vi "cRIO_4DoF_Admittance_controller_v3.vi"(0 "F":dbl[](array[numeric]), 1 "v_2 in":dbl[](array[numeric]), 2 "c":dbl[][](array[numeric])=[[1.0, 0.0, 0.0, 0.0], [0.0, 1.0, 0.0, 0.0], [0.0, 0.0, 1.0, 0.0], [0.0, 0.0, 0.0, 0.001]], 3 "m":dbl[][](array[numeric])=[[0.4, 0.0, 0.0, 0.0], [0.0, 0.4, 0.0, 0.0], [0.0, 0.0, 0.4, 0.0], [0.0, 0.0, 0.0, 0.0004]], 5 "Loop time (ms)":u32=10) -> (4 "del_m":dbl[](array[numeric]), 6 "v_2 out":dbl[][](array[numeric]))   [LabVIEW 2019]
uses:
  <vilib>/imath/engines/lvmath2/RunTimeEngine/BuiltInFunctions/inv/NIMS_inv(GM).vi
  <instcachedir>/0/NIMS_inv(GM)_A6DF8FE880224208AACFE4CF9F659502.lvgen/NIMS_inv(GM)_A6DF8FE880224208AACFE4CF9F659502_000.vi
  <vilib>/imath/engines/lvmath2/RunTimeEngine/ArithmeticOperatorToken/NIMS_ArithmeticOperator_multmx(M,CV).vi
  <instcachedir>/0/NIMS_ArithmeticOperator_multmx(M,CV)_1D61EED49E1847F3B05DBB8EDD2FBF8F.lvgen/NIMS_ArithmeticOperator_multmx(M,CV)_1D61EED49E1847F3B05DBB8EDD2FBF8F_000.vi
  <vilib>/imath/engines/lvmath2/RunTimeEngine/ArithmeticOperatorToken/NIMS_ArithmeticOperator_minus.vi
  <instcachedir>/0/NIMS_ArithmeticOperator_minus_12BFF9710EA5430A9EE87C5BC3F65186.lvgen/NIMS_ArithmeticOperator_minus_12BFF9710EA5430A9EE87C5BC3F65186_002.vi
  <vilib>/imath/engines/lvmath2/RunTimeEngine/ArithmeticOperatorToken/NIMS_ArithmeticOperator_multmx.vi
  <instcachedir>/0/NIMS_ArithmeticOperator_multmx_77F1D2D6F4D94BA7A97C4E7185C02392.lvgen/NIMS_ArithmeticOperator_multmx_77F1D2D6F4D94BA7A97C4E7185C02392_004.vi
  <vilib>/imath/engines/lvmath2/RunTimeEngine/ErrorHandling/NIMS_Create Error From Enums.vi
  <vilib>/imath/engines/lvmath2/RunTimeEngine/ArithmeticOperatorToken/NIMS_ArithmeticOperator_plus.vi
  <instcachedir>/0/NIMS_ArithmeticOperator_plus_5C9385B0197D46E2B844C41E02F9EC39.lvgen/NIMS_ArithmeticOperator_plus_5C9385B0197D46E2B844C41E02F9EC39_003.vi
  <vilib>/imathl/engines/lvmath/Functions/Error Handling/Create Error.vi
  <vilib>/imath/engines/lvmath2/RunTimeEngine/NodeEndStatement/NIMS_NodeEndStatement_Output.vi
  <instcachedir>/0/NIMS_NodeEndStatement_Output_53EC0D466D134D7ABD903AC30B43404B.lvgen/NIMS_NodeEndStatement_Output_53EC0D466D134D7ABD903AC30B43404B_002.vi
  <vilib>/imath/engines/lvmath2/RunTimeEngine/ErrorHandling/NIMS_Finalize Error.vi
panel:
  out "Waveform Chart":T1(graph)
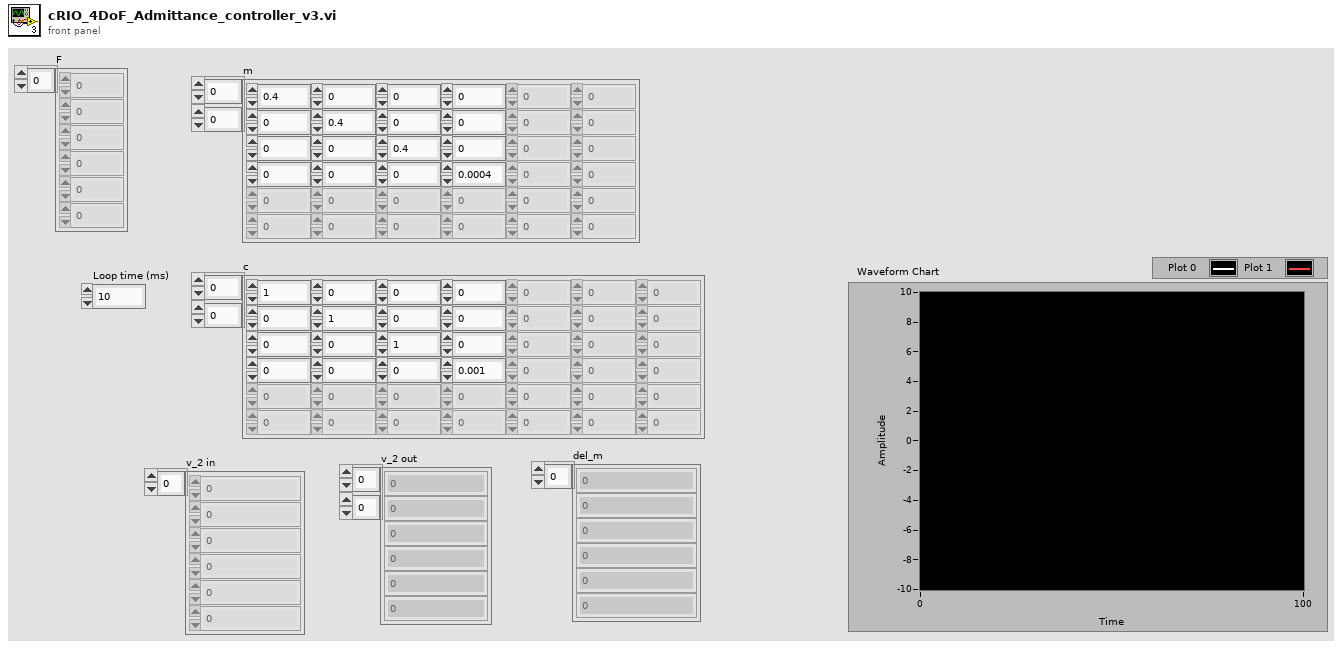
[diagram p1: front panel]
types:
  T1 = cluster{"del_m[0]":dbl, "del_m[1]":dbl, "del_m[2]":dbl, "del_m[3]":dbl, "del_m[4]":dbl, "del_m[5]":dbl, "del_m[6]":dbl, "del_m[7]":dbl, "del_m[8]":dbl}
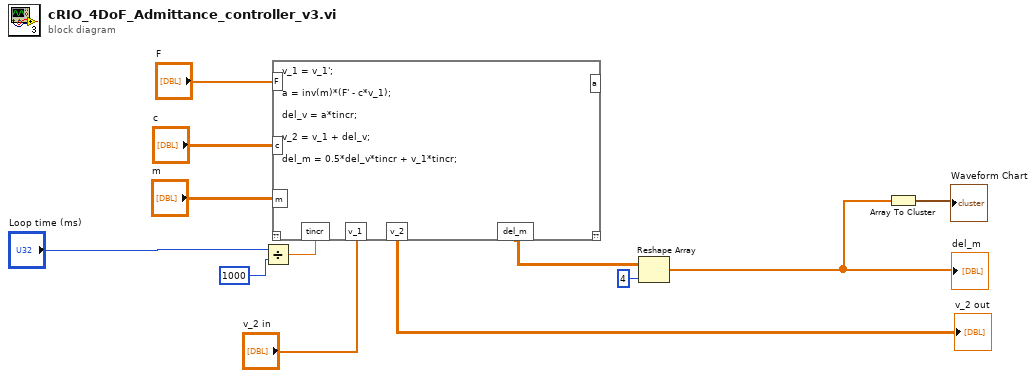
[diagram p0: block diagram]
diagram:
  n1 = Divide(x="Loop time (ms)", y=u32 1000 ("x")) -> (x/y=w12:dbl)
  n2 = mathscript code="v_1 = v_1';\n\na = inv(m)*(F' - c*v_1);\n\ndel_v = a*tincr;\n\nv_2 = v_1 + del_v;\n\ndel_m = 0.5*del_v*tincr + v_1*tincr;"("F"="F", "c"="c", "m"="m", "tincr"=w12, "v_1"="v_2 in") -> ("v_2"=→"v_2 out":dbl[][], "del_m"=w4:dbl[][])  [unwired: 1 in, 2 out]
  n3 = Reshape Array(w4, 4 ("dimension size")) -> (w2:dbl[])
  "del_m" <- w2
  n4 = Array To Cluster(array=w2) -> (cluster=→"Waveform Chart":T1)
